vi "MERGE DAQ and DAQmx .Sampling.Configure.vi"(8 "error in (no error)":errorcluster, 11 "Instrument.DAQ":refnum<class "Instrument.DAQ.lvclass">) -> (0 "error out":errorcluster, 2 "Restart Acquisition?":bool, 3 "Instrument.DAQ out":refnum<class "Instrument.DAQ.lvclass">)   [LabVIEW 2019, in "Instrument.Lockin.lvlib" / "Instrument.DAQ.lvclass"]
uses:
  Instrument.DAQ.lvclass
  Instrument.DAQ.lvclass/Instrument.DAQ.ctl
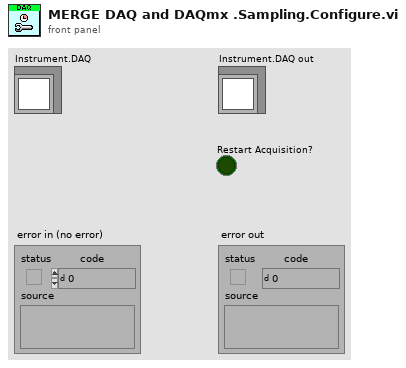
[diagram p1: front panel]
types:
  T1 = typedef "Instrument.Lockin.lvlib/Instrument.DAQ.lvclass/DAQ.Sampling--Cluster.ctl" = cluster{"Sampling":T2, "sample mode":i32, "Fs Mode":T3, "Fs Multiplier":dbl, "Refresh Rate (Hz)":dbl, "Decimation.PreDSP":i32, "Decimation.PostDSP":i32, "Fs.Output":dbl}
  T2 = typedef "Instrument.Lockin.lvlib/Instrument.DAQ.lvclass/DAQ.Sampling.Sampling--Cluster.ctl" = cluster{"Fs":dbl, "#s":i32}
  T3 = typedef "Instrument.Lockin.lvlib/Instrument.DAQ.lvclass/DAQ.Sampling.Fs Mode--enum.ctl" = enum16{"Manual", "Auto Fs", "Max Fs"}
  T4 = cluster{"Sampling":cluster{"Fs":bool, "#s":bool}, "sample mode":bool, "Fs Mode":bool, "Fs Multiplier":bool, "Refresh Rate (Hz)":bool, "Decimation.PreDSP":bool, "Decimation.PostDSP":bool, "Fs.Output":bool}
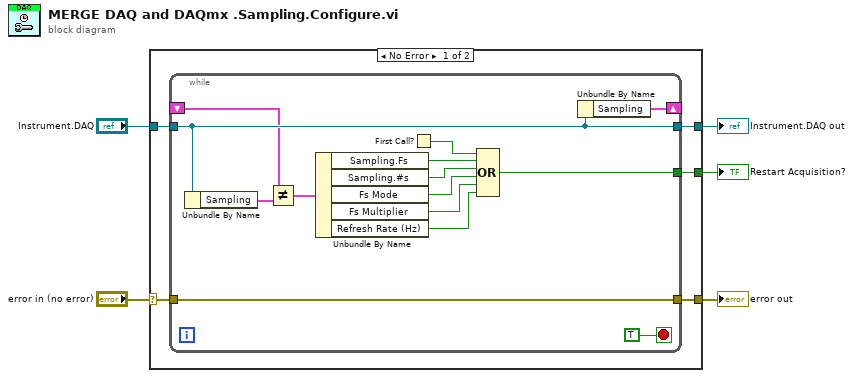
[diagram p0: block diagram]
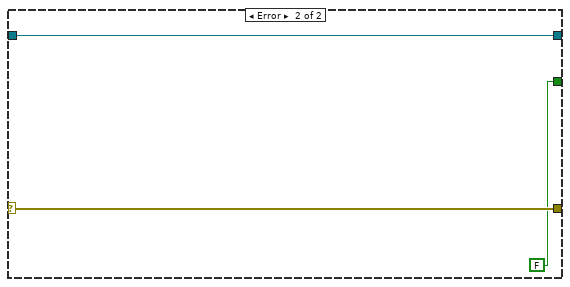
[diagram p2: hidden frame]
diagram:
  n1 = case shown="No Error" "error in (no error)" {
    selector: "error in (no error)" -> [w9 w27]
    tunnel: "Instrument.DAQ" -> [w10 w26]
    tunnel: [w6 w26] -> w3
    tunnel: [w8 w27] -> w2
    tunnel: [w7 FALSE] -> w1
    frame No Error {
      n2 = while {
        tunnel: [w13] -> w7
        tunnel: w10 -> [w21]
        tunnel: [w21] -> w6
        tunnel: w9 -> [w22]
        tunnel: [w22] -> w8
        shift-right: [w23] -> _
        shift-left: _ -> [w11]
        stop <- TRUE stop-if-true
        n3 = Unbundle By Name(w21) -> ("Sampling"=w12:T1)
        n4 = Not Equal?(x=w11, y=w12) -> (x != y?=w14:T4)
        n5 = Unbundle By Name(w14) -> ("Sampling.Fs"=w20:bool, "Sampling.#s"=w19:bool, "Fs Mode"=w18:bool, "Fs Multiplier"=w17:bool, "Refresh Rate (Hz)"=w16:bool)
        n6 = First Call?() -> (First Call?: T/F=w15:bool)
        n7 = Compound Arithmetic op=OR(w15, w20, w19, w18, w17, w16) -> (w13:bool)
        n8 = Unbundle By Name(w21) -> ("Sampling"=w23:T1)
      }
    }
    frame Error {
    }
  }
  "Instrument.DAQ out" <- w3
  "error out" <- w2
  "Restart Acquisition?" <- w1
